vi "RTD Temp.vi"(2 "error in (no error)":errorcluster, 3 "DAQmx Physical Channel":tag) -> (0 "error out":errorcluster, 1 "RTD Temp":dbl(slide) scale=0.0..100.0)   [LabVIEW 2021]
doc: "Toma 10 muestras de temperatura del canal de la DAQ pasado como input,les hace la media y devuelve un valor de temperatura donde se compensa el posible ruido."
uses:
  <vilib>/DAQmx/read.llb/DAQmx Read (Analog 1D DBL 1Chan NSamp).vi
  <vilib>/Analysis/baseanly.llb/Mean (DBL).vi
  <vilib>/DAQmx/create/channels.llb/DAQmx Create Channel (AI-Voltage-Basic).vi
  <vilib>/DAQmx/configure/timing.llb/DAQmx Timing (Sample Clock).vi
  <vilib>/DAQmx/miscellaneous.llb/DAQmx Fill In Error Info.vi
  <vilib>/Analysis/NI_AALBase.lvlib
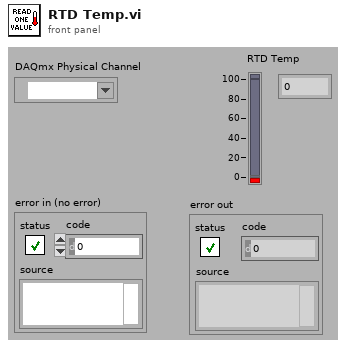
[diagram p1: front panel]
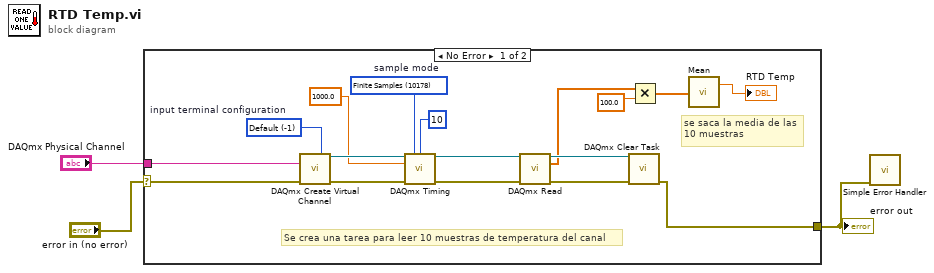
[diagram p0: block diagram]
diagram:
  n1 = case shown="No Error" "error in (no error)" {
    selector: "error in (no error)" -> [w20 w21]
    tunnel: [w16 w21] -> w2
    tunnel: "DAQmx Physical Channel" -> [w15 _]
    frame No Error {
      w4 = -1 items=["Default"=-1, "RSE"=10083, "NRSE"=10078, "Differential"=10106, "Pseudodifferential"=12529]  # input terminal configuration
      w6 = 10178 items=["Finite Samples"=10178, "Continuous Samples"=10123, "Hardware Timed Single Point"=12522]  # sample mode
      # "se saca la media de las\n10 muestras"
      # "Se crea una tarea para leer 10 muestras de temperatura del canal"
      n2 = call-poly <vilib>:"DAQmx Create Virtual Channel.vi"("input terminal configuration"=w4, "physical channels"=w15, "error in"=w20) -> ("task out"=w14:refnum<k21>, "error out"=w19:errorcluster)  [unwired: 11 in]
      n3 = call-poly <vilib>:"DAQmx Timing.vi"("task/channels in"=w14, "sample mode"=w6, "samples per channel"=10, "rate"=1000.0, "error in"=w19) -> ("task out"=w13:refnum<k21>, "error out"=w18:errorcluster)  [unwired: 9 in]
      n4 = call-poly <vilib>:"DAQmx Read.vi"("task/channels in"=w13, "error in"=w18) -> ("task out"=w12:refnum<k21>, "data"=w11:dbl[], "error out"=w17:errorcluster)  [unwired: 11 in]
      n5 = call <vilib>:"DAQmx Clear Task.vi"("task in"=w12, "error in"=w17) -> ("error out"=w16:errorcluster)  [unwired: 13 in]
      n6 = Multiply(x=w11, y=100.0) -> (x*y=w9:dbl[])
      n7 = call-poly <vilib>:"Mean.vi"("X"=w9) -> ("mean"=→"RTD Temp":dbl)  [unwired: 1 out]
    }
    frame Error {
    }
  }
  "error out" <- w2
  n8 = call <vilib>:"Simple Error Handler.vi"("error in (no error)"=w2) -> ()  [unwired: 4 in, 5 out]
